vi "VisionBegin.vi"(8 "error in (no error)":errorcluster) -> (0 "error out":errorcluster)   [LabVIEW 2023]
doc: "Begin for vision\n\nInputs:\n -- Error in -- Error cluster -- propagated error input\n\nOutputs:\n -- Error out -- Error cluster -- progated error output"
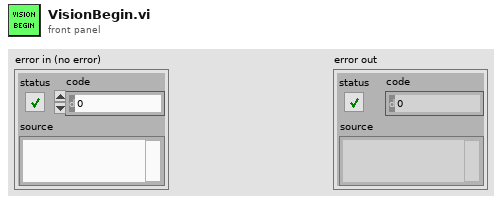
[diagram p1: front panel]
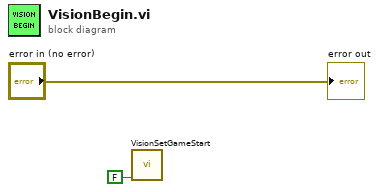
[diagram p0: block diagram]
diagram:
  n1 = call "VisionSetGameStart.vi"("Game Start"=FALSE) -> ()  [unwired: 11 in]
  "error out" <- "error in (no error)"
